vi "Read Measured Amplitude.vi"(8 "error in (no error)":errorcluster, 11 "Measure Waveform in":refnum<class "Measure Waveform.lvclass">) -> (0 "error out":errorcluster, 2 "Abs_Double Float.lvclass":refnum<class "Abs_Double Float.lvclass">, 3 "Measure Waveform out":refnum<class "Measure Waveform.lvclass">)   [LabVIEW 2021, in "Measure Waveform.lvclass"]
uses:
  Measure Waveform.lvclass
  <vilib>/TSA/Abstract Data Classes/Abs_Types/Double Float/Abs_Double Float.lvclass
  Measure Waveform.lvclass/Measure Waveform.ctl
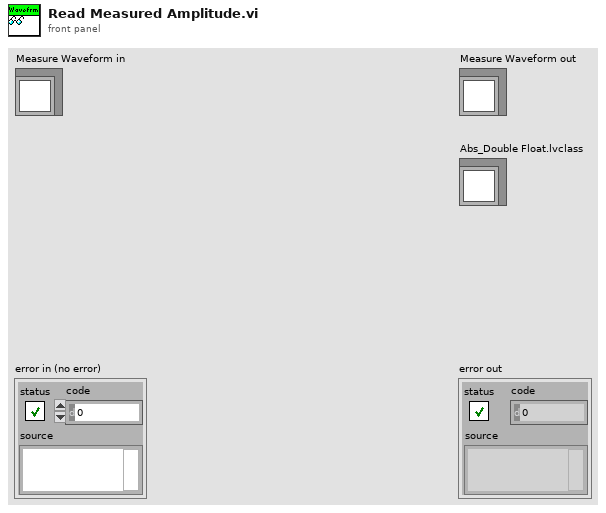
[diagram p1: front panel]
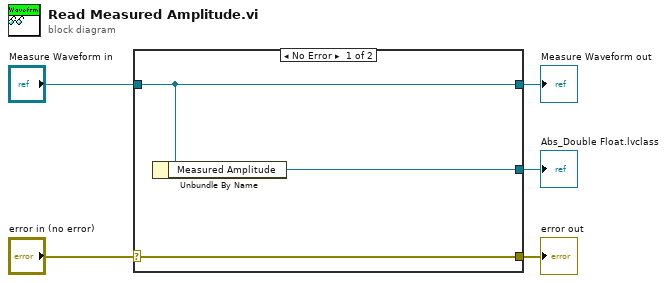
[diagram p0: block diagram]
diagram:
  n1 = case shown="No Error" "error in (no error)" {
    selector: "error in (no error)" -> [w8 w9]
    tunnel: [w8 w9] -> w4
    tunnel: [w7 w10] -> w2
    tunnel: "Measure Waveform in" -> [w7 w10]
    tunnel: [w6 _] -> w1
    frame No Error {
      n2 = Unbundle By Name(w7) -> ("Measured Amplitude"=w6:refnum<class "Abs_Double Float.lvclass">)
    }
    frame Error {
    }
  }
  "error out" <- w4
  "Measure Waveform out" <- w2
  "Abs_Double Float.lvclass" <- w1
